vi "Hello World.vi"() -> ()   [LabVIEW 2024]
panel:
  in  "message":string="This is my first VI"
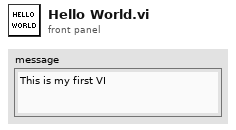
[diagram p1: front panel]
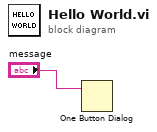
[diagram p0: block diagram]
diagram:
  n1 = One Button Dialog(message="message") -> ()  [unwired: 1 in, 1 out]
